vi "Protocol Write.vi"(8 "error in (no error)":errorcluster, 10 "data":u8[](array[numeric]), 11 "protocol layer in":refnum<class "TCP.lvclass">) -> (0 "error out":errorcluster, 1 "timed out?":bool, 3 "protocol layer out":refnum<class "TCP.lvclass">)   [LabVIEW 2019, in "TCP.lvclass"]
doc: "Writes to the established TCP connection stored in the class."
uses:
  TCP.lvclass
  TCP.lvclass/TCP.ctl
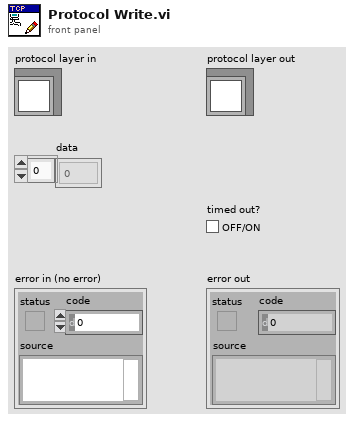
[diagram p1: front panel]
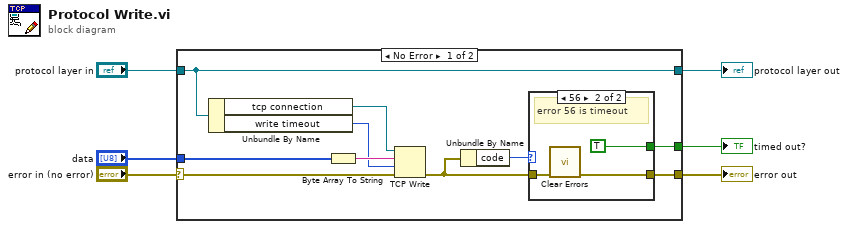
[diagram p0: block diagram]
diagram:
  n1 = case shown="No Error" "error in (no error)" {
    selector: "error in (no error)" -> [w12 w22]
    tunnel: [w16 w22] -> w4
    tunnel: "data" -> [w15 _]
    tunnel: [w10 _] -> w3
    tunnel: "protocol layer in" -> [w8 w21]
    tunnel: [w8 w21] -> w1
    frame No Error {
      n2 = Unbundle By Name(w8) -> ("tcp connection"=w9:refnum<k5>, "write timeout"=w7:i32)
      n3 = Byte Array To String(unsigned byte array=w15) -> (string=w14:string)
      n4 = TCP Write(connection ID=w9, data in=w14, error in (no error)=w12, 9:w7) -> (error out=w13:errorcluster)  [unwired: 2 out]
      n5 = Unbundle By Name(w13) -> ("code"=w11:i32)
      n6 = case shown="56" w11 {
        tunnel: w13 -> [w17 w19]
        tunnel: [w17 w18] -> w16
        tunnel: [_ TRUE] -> w10
        frame 0, Default {
        }
        frame 56 {
          # "error 56 is timeout"
          n7 = call <vilib>:"Clear Errors.vi"("error in (no error)"=w19) -> ("error out"=w18:errorcluster)  [unwired: 5 in, 1 out]
        }
      }
    }
    frame Error {
    }
  }
  "error out" <- w4
  "protocol layer out" <- w1
  "timed out?" <- w3
